vi "LVClass_SlopesPostProcessList GetParameter_Filter.vi"(0 "SlopesPostProcessorList in":refnum<class "SlopesPostProcessorList.lvclass">, 5 "Position":u32, 11 "error in (no error)":errorcluster) -> (4 "SlopesPostProcessorList out":refnum<class "SlopesPostProcessorList.lvclass">, 8 "filter":T1, 15 "error out":errorcluster)   [LabVIEW 2020, in "SlopesPostProcessorList.lvclass"]
doc: "Get parameters of the Filter processor.\n\n--------------------------------------------------------------------------------\n\n<B>SlopesPostProcessorListIn </B> : SlopesPostProcessorList object.\n<B>SlopesPostProcessorListOut </B> : SlopesPostProcessorList object.\n<B>position </B> : Position of the processor in the SlopesPostProcessorList.\n<B>is_tiltx_filter_on </B> : X tilt filter state.\n<B>is_tilty_filter_on </B> : Y tilt filter state.\n<B>is_curv_filter_on </B> : Curvature filter state.\n<B>is_astig0_filter_on </B> : 0 degree astigmatism filter state.\n<B>is_astig45_filter_on </B> : 45 degree astigmatism filter state.\n<B>is_others_filter_on </B> : All other aberrations filter state.\n<B>ErrorIn </B> : Error\n<B>ErrorOut </B> : Error\n\n--------------------------------------------------------------------------------"
uses:
  SlopesPostProcessorList.lvclass
  Controls/SlopesPostProcessorList - Filter.ctl
  SlopesPostProcessorList.lvclass/SlopesPostProcessorList.ctl
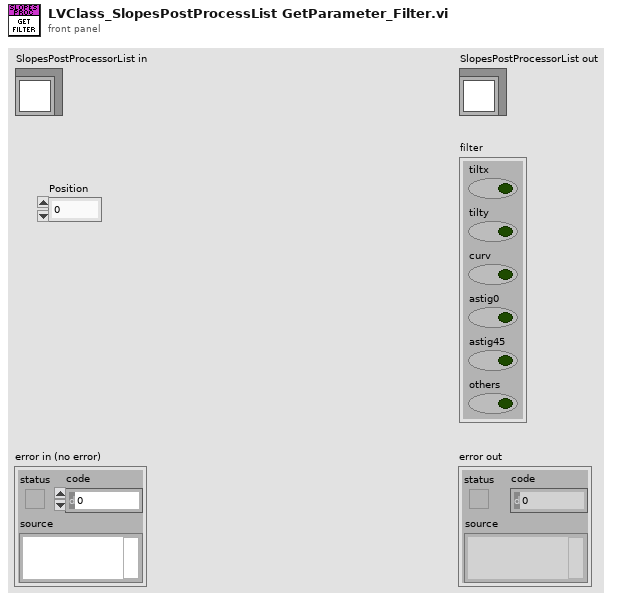
[diagram p1: front panel]
types:
  T1 = typedef "SlopesPostProcessorList - Filter.ctl" = cluster{"tiltx":bool, "tilty":bool, "curv":bool, "astig0":bool, "astig45":bool, "others":bool}
  T2 = typedef "ClassID.ctl" = i64
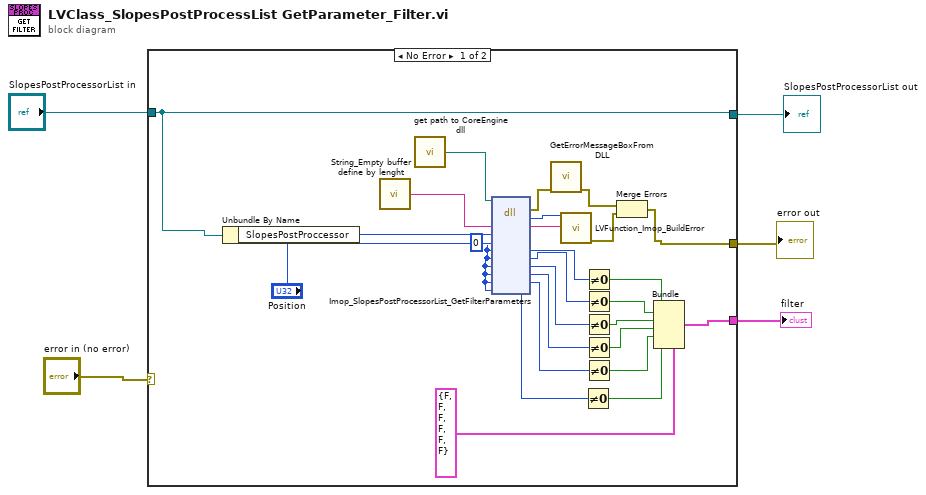
[diagram p0: block diagram]
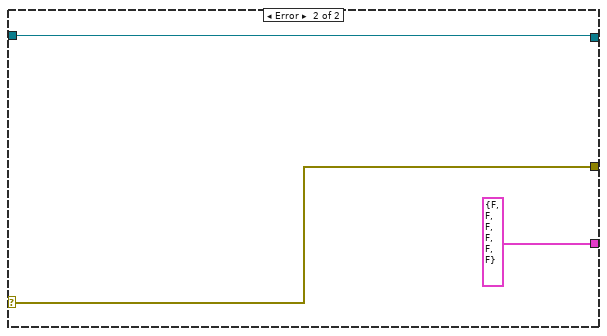
[diagram p2: hidden frame]
diagram:
  n1 = case shown="No Error" "error in (no error)" {
    selector: "error in (no error)" -> [_ w33]
    tunnel: "SlopesPostProcessorList in" -> [w26 w34]
    tunnel: [w26 w34] -> w3
    tunnel: [w10 w33] -> w2
    tunnel: [w13 T1 {"tiltx"=FALSE, "tilty"=FALSE, "curv"=FALSE, "astig0"=FALSE, "astig45"=FALSE, "others"=FALSE} ("filter")] -> w1
    frame No Error {
      w8 = u8 0 ("tiltx")
      n2 = Unbundle By Name(w26) -> ("SlopesPostProccessor"=w25:T2)
      n3 = call "String_Empty buffer define by lenght.vi"() -> ("Empty buffer"=w31:string)  [unwired: 1 in]
      n4 = call "get path to CoreEngine dll.vi"() -> ("path to wavekit library"=w28:path)  [unwired: 14 in, 1 out]
      n5 = dll-call lib="D:/soft/HASO_v3/SVN_trunk/ImOpCoreEngine4_LV2011/DLLs/c_interface_vc100.dll" fn="Imop_SlopesPostProcessorList_GetFilterParameters"(path in=w28, "message"=w31, "objet"=w25, "Position"="Position", "tiltx"=w8, "tilty"=w8, "curv"=w8, "astig0"=w8, "astig45"=w8, "others"=w8) -> (error out=w27:errorcluster, "return type"=w29:i32, "message"=w30:string, "tiltx"=w24:u8, "tilty"=w23:u8, "curv"=w22:u8, "astig0"=w21:u8, "astig45"=w20:u8, "others"=w9:u8)  [unwired: 4 in, 1 out]
      n6 = call "GetErrorMessageBoxFromDLL.vi"("error IN"=w27) -> ("error OUT"=w12:errorcluster)  [unwired: 10 in]
      n7 = call "LVFunction_Imop_BuildError.vi"("code"=w29, "String to Prepend to source (\"\")"=w30) -> ("error out"=w11:errorcluster)  [unwired: 13 in]
      n8 = Not Equal To 0?(x=w9) -> (x != 0?=w6:bool)
      n9 = Not Equal To 0?(x=w24) -> (x != 0?=w18:bool)
      n10 = Not Equal To 0?(x=w23) -> (x != 0?=w17:bool)
      n11 = Not Equal To 0?(x=w22) -> (x != 0?=w16:bool)
      n12 = Not Equal To 0?(x=w21) -> (x != 0?=w15:bool)
      n13 = Not Equal To 0?(x=w20) -> (x != 0?=w14:bool)
      n14 = Merge Errors(w12, w11) -> (w10:errorcluster)
      n15 = Bundle(cluster=T1 {"tiltx"=FALSE, "tilty"=FALSE, "curv"=FALSE, "astig0"=FALSE, "astig45"=FALSE, "others"=FALSE} ("filter"), "tiltx"=w18, "tilty"=w17, "curv"=w16, "astig0"=w15, "astig45"=w14, "others"=w6) -> (w13:T1)
    }
    frame Error {
    }
  }
  "error out" <- w2
  "SlopesPostProcessorList out" <- w3
  "filter" <- w1
